vi "Amplitude modulation.vi"() -> ()   [LabVIEW 2018]
panel:
  in  "carrier frequency":dbl(knob) scale=0.0..100.0
  out "Modulated wave":dynamicdata(graph)
  out "carrier signal":dynamicdata(graph)
  out "Messenger signal":dynamicdata(graph)
  in  "stop":bool
  in  "Modulation index":dbl(knob) scale=0.0..1.0
  in  "message frequency":dbl(knob) scale=0.0..100.0
  # "170040320 - 15"
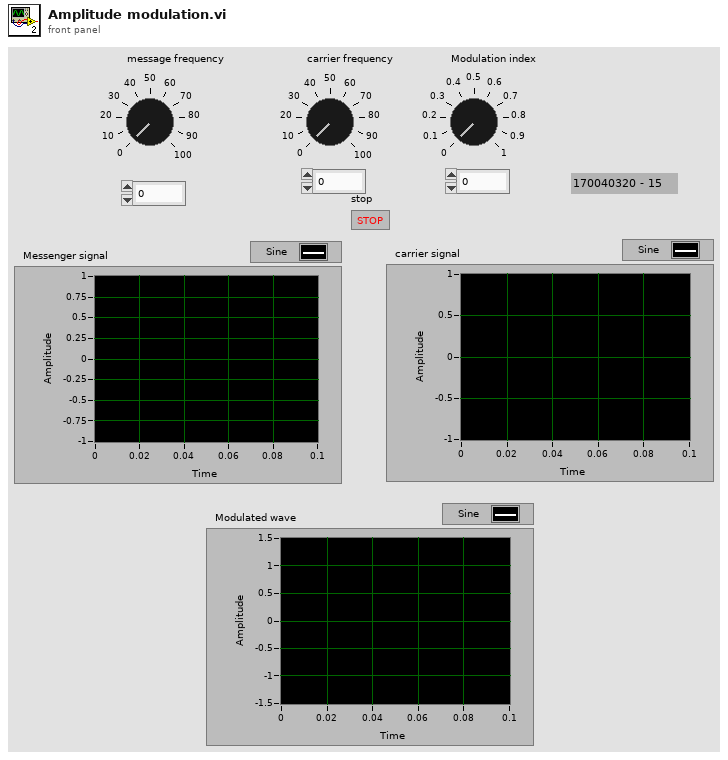
[diagram p1: front panel]
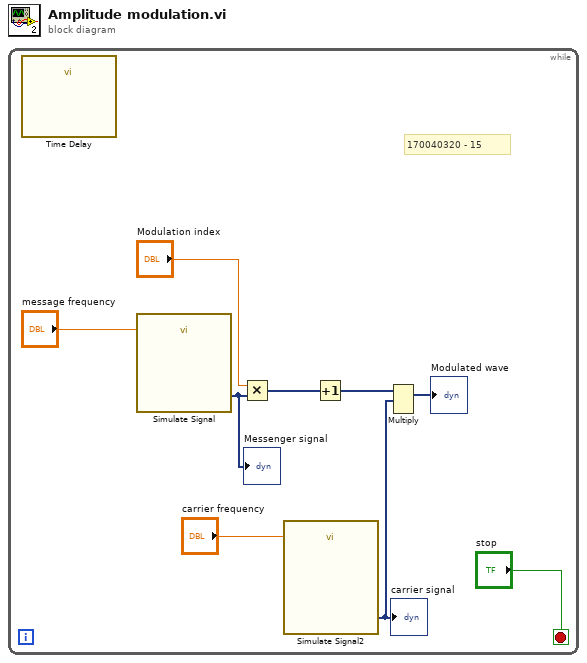
[diagram p0: block diagram]
diagram:
  n1 = while {
    stop <- "stop" stop-if-true
    # "170040320 - 15"
    n2 = call "Time Delay"() -> ()  [unwired: 11 in, 1 out]
    n3 = call "Simulate Signal"("Frequency"="message frequency") -> ("Sine"=w3:dynamicdata)  [unwired: 13 in, 1 out]
    "Messenger signal" <- w3
    n4 = Multiply(x="Modulation index", y=w3) -> (x*y=w9:dynamicdata)
    n5 = call "Simulate Signal2"("Frequency"="carrier frequency") -> ("Sine"=w7:dynamicdata)  [unwired: 13 in, 1 out]
    "carrier signal" <- w7
    n6 = Increment(x=w9) -> (x+1=w8:dynamicdata)
    n7 = Multiply(1:w7, 2:w8) -> (0:→"Modulated wave":dynamicdata)  [unwired: 1 in, 1 out]
  }
